vi "ReadOutputPathRequest.vi"(8 "error in (no error)":errorcluster, 11 "ModuleID":i32) -> (0 "error out":errorcluster)   [LabVIEW 2014, in "OutputToFileModule.lvlib"]
uses:
  OutputToFileModule.lvlib
  Private/clEventType.ctl
  <vilib>/Utility/error.llb/Error Cluster From Error Code.vi
  <vilib>/ErrorRing/Error Ring.xnode
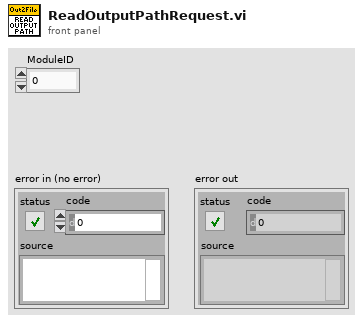
[diagram p1: front panel]
types:
  T1 = typedef "OutputToFileModule.lvlib/clRequestEvents.ctl" = cluster{"StopRequest":refnum<user-event>, "LoadPluginRequest":refnum<user-event>, "ReadPathToPluginRequest":refnum<user-event>, "WriteEvtRptRequest":refnum<user-event>, "WritePmuImpairRptRequest":refnum<user-event>, "WriteNetTimeRequest":refnum<user-event>, "WritePktLossRequest":refnum<user-event>, "WritePmuConfigRequest":refnum<user-event>, "ReadPmuConfigRequest":refnum<user-event>, "WriteOutPathRequest":refnum<user-event>, "ReadOutPathRequest":refnum<user-event>, "WriteFlagImpairRequest":refnum<user-event>, "OutputRefFileRequest":refnum<user-event>, "OutputImpairedFileRequest":refnum<user-event>, "OutputErrorDataRequest":refnum<user-event>, "OpenConfigRequest":refnum<user-event>, "ShowPanel":refnum<user-event>}
  T2 = typedef "OutputToFileModule.lvlib/clEventType.ctl" = cluster{"ModuleID":i32, "Data":variant}
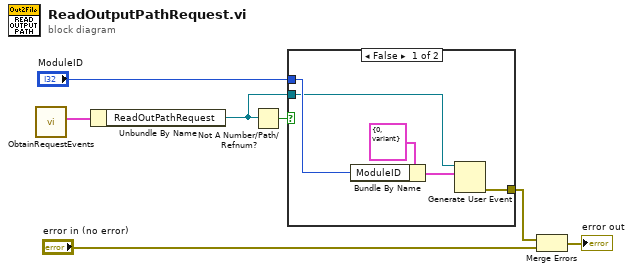
[diagram p0: block diagram]
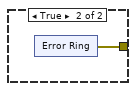
[diagram p2: hidden frame]
diagram:
  n1 = call "ObtainRequestEvents.vi"() -> ("clRequestEvents"=w7:T1)  [unwired: 10 in, 1 out]
  n2 = Unbundle By Name(w7) -> ("ReadOutPathRequest"=w4:refnum<user-event>)
  n3 = Not A Number/Path/Refnum?(number/path/refnum=w4) -> (NaN/Path/Refnum?=w6:bool)
  n4 = case shown="False" w6 {
    tunnel: "ModuleID" -> [w11 _]
    tunnel: w4 -> [w10 _]
    tunnel: [w8 w13] -> w3
    frame False {
      n5 = Bundle By Name(cluster=T2 {"ModuleID"=0, "Data"=variant} ("clEventType"), "ModuleID"=w11) -> (w9:T2)
      n6 = Generate User Event(user event=w10, event data cluster=w9) -> (error out=w8:errorcluster)  [unwired: 2 in, 1 out]
    }
    frame True {
      n7 = xnode "Error Ring"() -> ("error out"=w13:errorcluster)
    }
  }
  n8 = Merge Errors(w3, "error in (no error)") -> (→"error out":errorcluster)
